vi "YOKOGAWA_CSU-X1.vi"() -> ()   [LabVIEW 2024]
uses:
  States_Ctl.ctl
  <vilib>/Instr/_visa.llb/VISA Flush IO Buffer Mask.ctl
  <vilib>/Instr/_visa.llb/VISA Configure Serial Port (Instr).vi
panel:
  out "YOKOGAWA COM PORT":refnum<visa-resource-name>
  out "Current DM name":string
  out "Current DM position":u16 min=1 max=3 step=1
  out "Current rotation speed":u16=5000 min=1 max=3 step=1
  out "Current filter name 2":string="647LP"
  out "Current Filter position 2":u16=6 min=1 max=3 step=1
  out "Current filter name":string="647LP"
  out "Current Filter position":u16=6 min=1 max=3 step=1
  out "Number of Open/Close":i32=73
  in  "DM names":string[](array[string])=["405488568647", "445514593"]
  in  "DM position":u8=1 min=1 max=2 step=1
  in  "Filter names 2":string[](array[string])=["447BP60", "475BP35", "525BP50", "600BP37", "647BP57", "647LP"]
  in  "FW Position 2":u8=6 min=1 max=6 step=1
  in  "FW Speed 2":u8=3 min=1 max=3 step=1
  in  "Filter names 1":string[](array[string])
  in  "FW Position 1":u8=6 min=1 max=6 step=1
  in  "FW Speed 1":u8=2 min=1 max=3 step=1
  in  "Exposure time (ms)":dbl=50.0 max=5000.0 step=100.0
  in  "Adjust rotation speed\nto exposure time?":bool
  in  "Disk Speed (rpm)":u16=5000 max=0 step=100
  in  "Rotation?":bool=TRUE
  in  "Save dichroic mirror names":bool
  in  "Save filter names":bool
  in  "Shutter":bool
  out "error out":errorcluster
  in  "error in (no error)":errorcluster
  in  "STOP":bool
  # "Disk"
  # "Filter wheel 1"
  # "Filter wheel 2"
  # "Dichroic mirror"
  # "General"
  # "Status"
  # "Advanced settings"
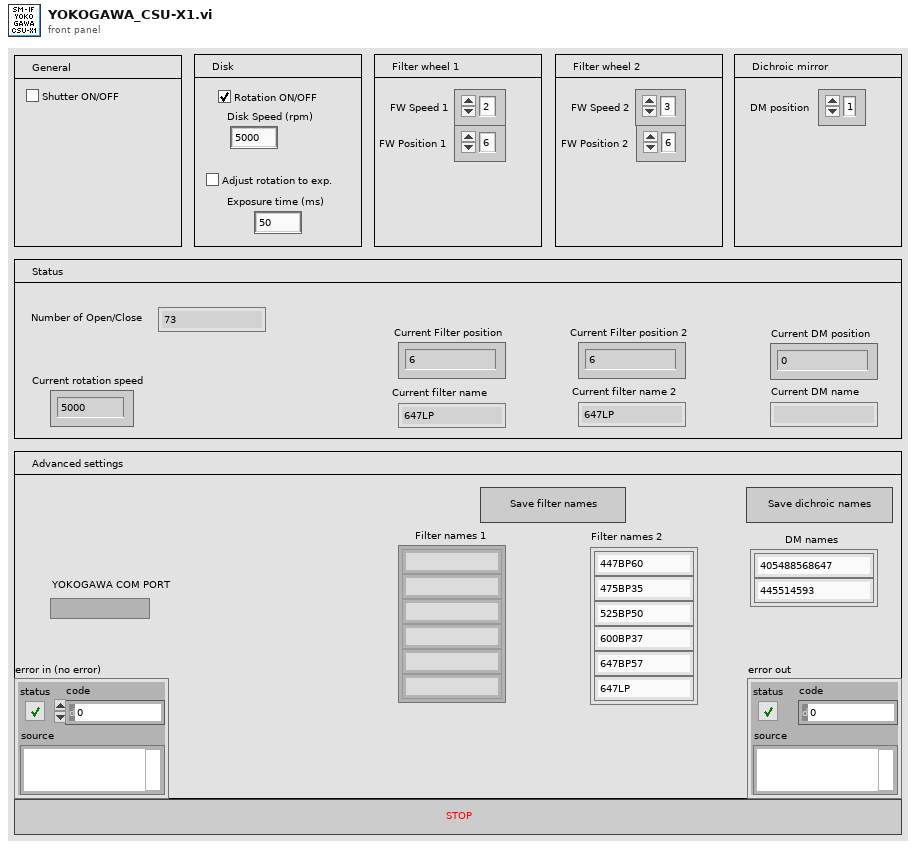
[diagram p1: front panel]
types:
  T1 = typedef "States_Ctl.ctl" = enum16{"INITIALIZE", "WRITE_COMMAND", "CHECK_SHUTTER_STATUS", "CHECK_SHUTTER_COUNT", "CHECK_DISK_SPEED", "CHECK_MAX_DISK_SPEED", "CHECK_FILTER_NAMES", "CHECK_FW_POSITION", "CHECK_DM_POSITION", "CHECK_DM_NAMES", "EXIT"}
  T2 = typedef "VISA Flush IO Buffer Mask.ctl" = u16
  T3 = cluster{"State":T1, "YOKOGAWA COM PORT":refnum<visa-resource-name>}
  T4 = cluster{"State":T1, "Dichroic mirror position":u8}
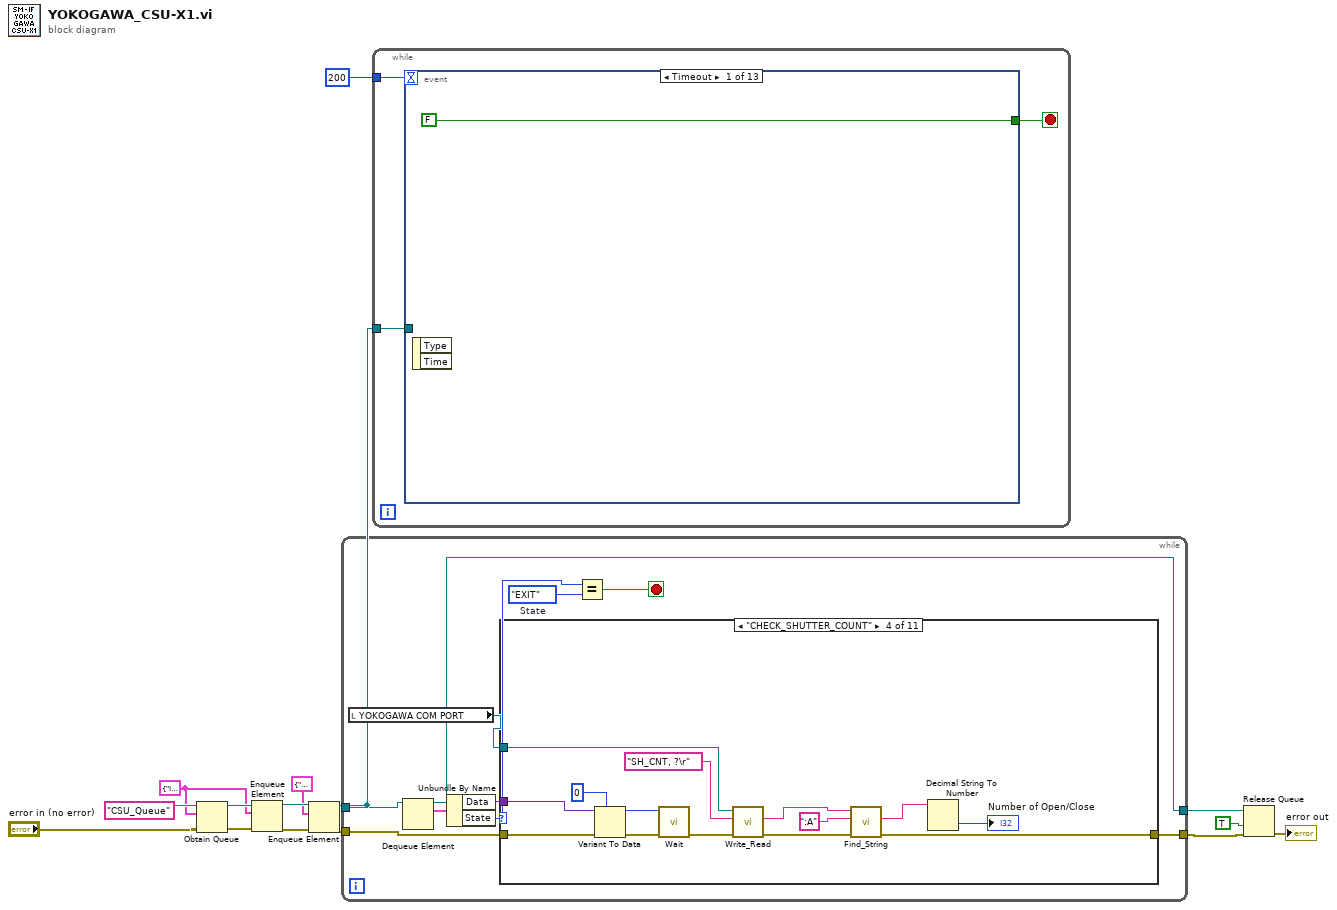
[diagram p0: block diagram]
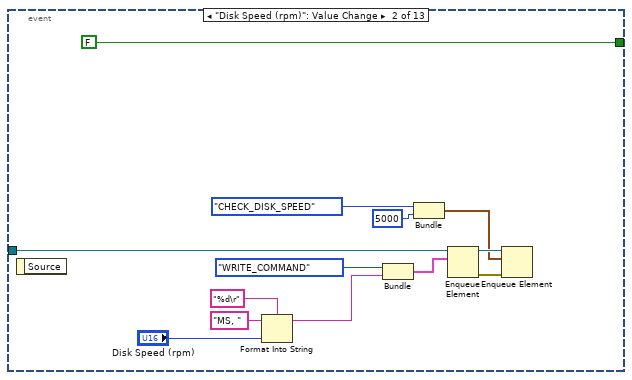
[diagram p2: hidden frame]
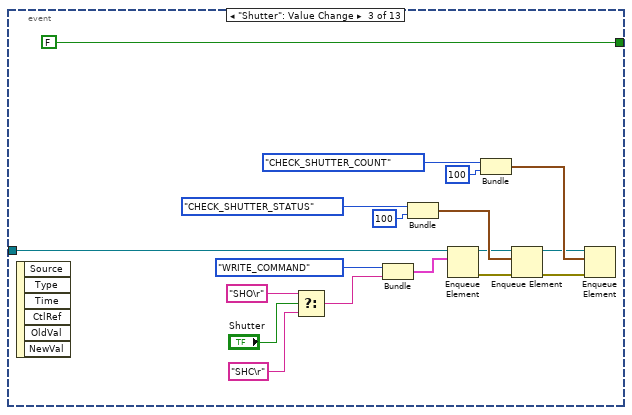
[diagram p3: hidden frame]
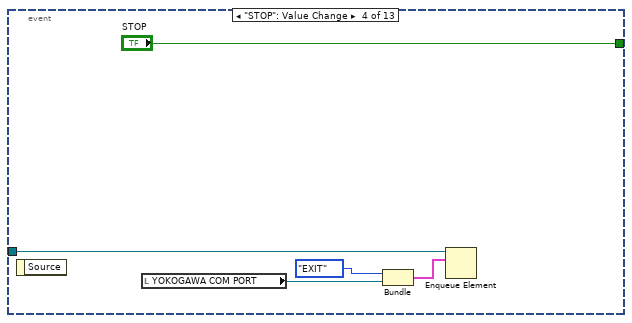
[diagram p4: hidden frame]
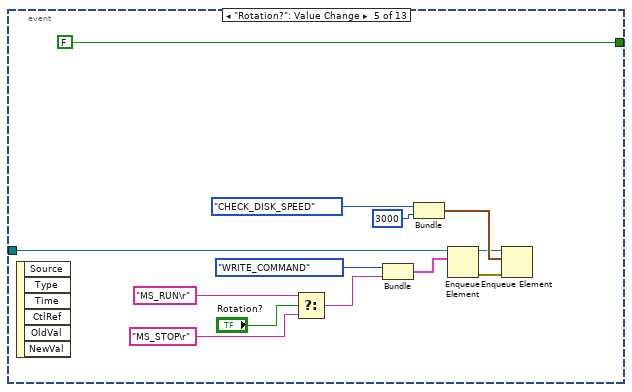
[diagram p5: hidden frame]
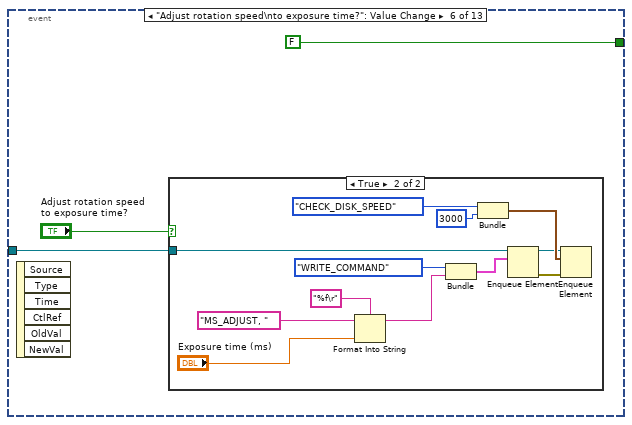
[diagram p6: hidden frame]
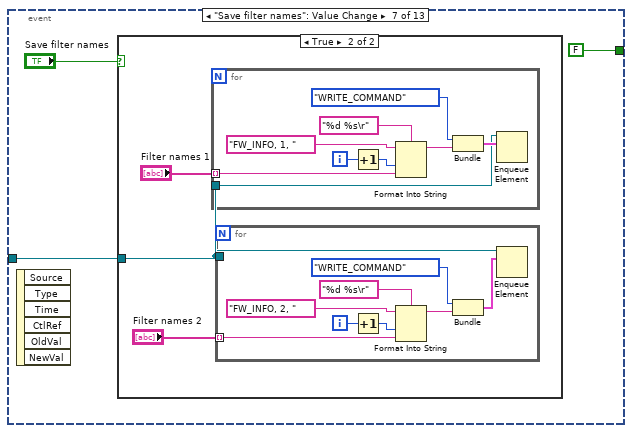
[diagram p8: hidden frame]
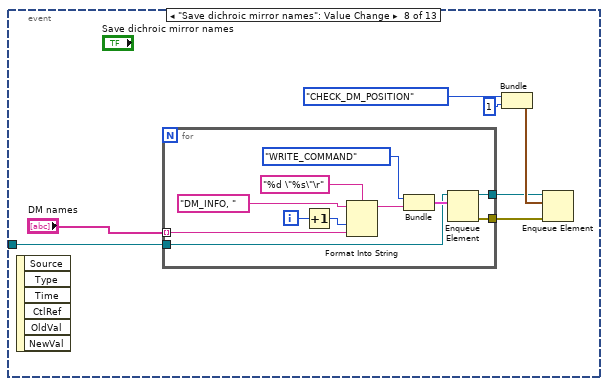
[diagram p10: hidden frame]
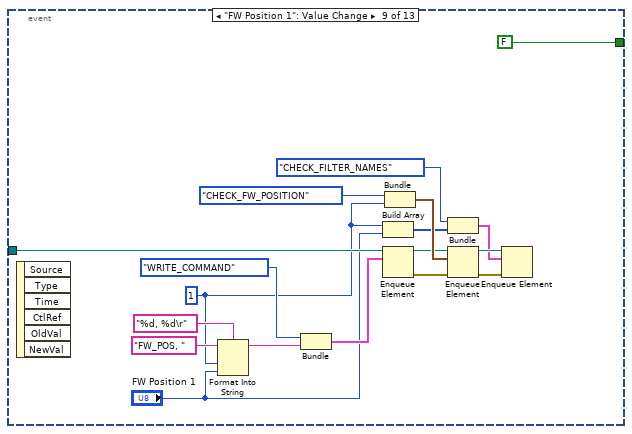
[diagram p11: hidden frame]
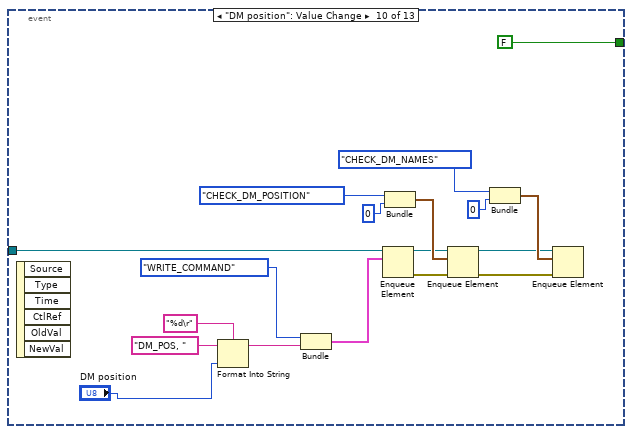
[diagram p12: hidden frame]
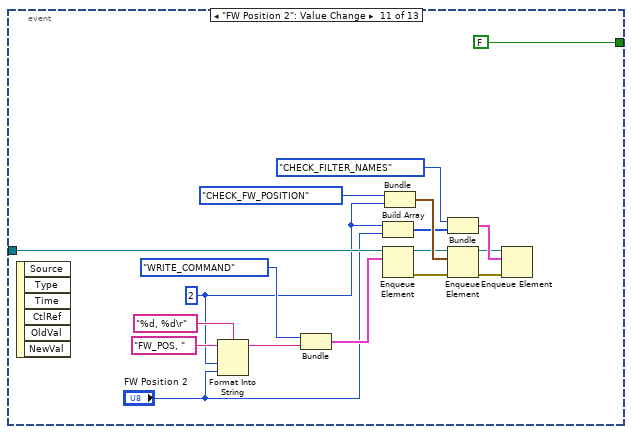
[diagram p13: hidden frame]
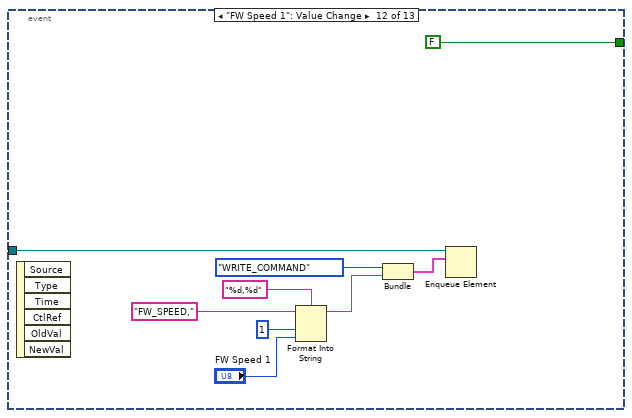
[diagram p14: hidden frame]
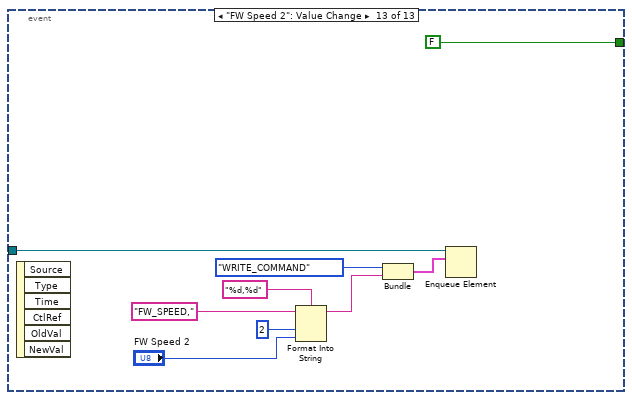
[diagram p15: hidden frame]
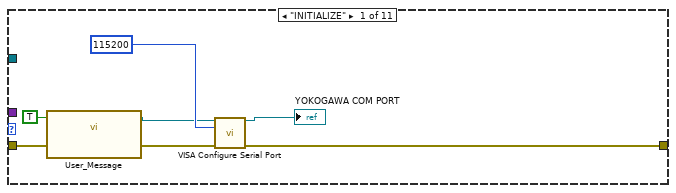
[diagram p16: hidden frame]
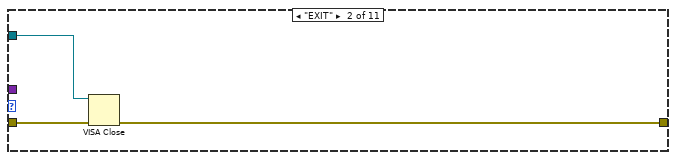
[diagram p17: hidden frame]
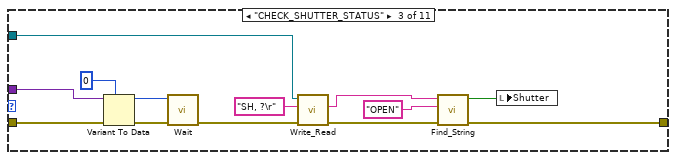
[diagram p18: hidden frame]
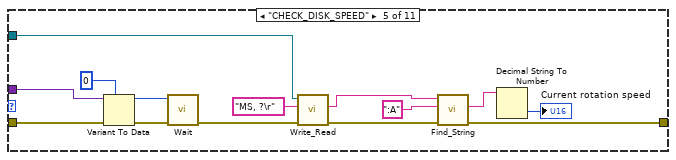
[diagram p19: hidden frame]
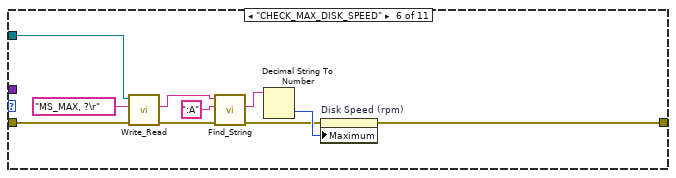
[diagram p20: hidden frame]
diagram:
  w12 = cluster{"State":T1, "Data":variant} {"State"=enum."INITIALIZE", "Data"=variant} ("cluFNData")
  n1 = Obtain Queue(name (unnamed)="CSU_Queue", element data type=w12, error in (no error)="error in (no error)") -> (queue out=w13:refnum<queue>, error out=w14:errorcluster)  [unwired: 2 in, 1 out]
  n2 = Enqueue Element(queue=w13, element=w12, error in (no error)=w14) -> (queue out=w7:refnum<queue>, error out=w8:errorcluster)  [unwired: 1 in, 1 out]
  n3 = Enqueue Element(queue=w7, element=cluster{"State":T1, "Data":variant} {"State"=enum."CHECK_MAX_DISK_SPEED", "Data"=variant} ("cluFNData"), error in (no error)=w8) -> (queue out=w1:refnum<queue>, error out=w5:errorcluster)  [unwired: 1 in, 1 out]
  n4 = while {
    tunnel: w5 -> [w21]
    tunnel: w1 -> [w20]
    tunnel: [w19] -> w4
    tunnel: [w18] -> w3
    stop <- w17 stop-if-true
    w22 = States_Ctl."EXIT"  # State
    n5 = local read "YOKOGAWA COM PORT"() -> (w16:refnum<visa-resource-name>)
    n6 = Dequeue Element(queue=w20) -> (queue out=w19:refnum<queue>, element=w23:cluster{"State":T1, "Data":variant})  [unwired: 2 in, 2 out]
    n7 = Unbundle By Name(w23) -> ("Data"=w24:variant, "State"=w25:T1)
    n8 = case shown="\"CHECK_SHUTTER_COUNT\"" w25 {
      tunnel: w21 -> [w30 w34 w37 w50 w65 w81 w91 w108 w123 w150 w156]
      tunnel: [w31 w35 w43 w56 w71 w77 w92 w102 w128 w137 w158] -> w18
      tunnel: w24 -> [_ _ w36 w51 w64 _ w94 w109 _ w151 _]
      tunnel: w16 -> [_ w33 w42 w57 w69 w80 w90 w110 w121 w142 w157]
      frame "INITIALIZE" {
        n9 = call "User_Message.vi"("Enable"=TRUE, "error in (no error)"=w30) -> ("CSU COM PORT  2"=w26:refnum<visa-resource-name>, "error out"=w28:errorcluster)  [unwired: 15 in, 1 out]
        n10 = call-poly "VISA Configure Serial Port"("VISA resource name"=w26, "baud rate (9600)"=u32 115200, "error in (no error)"=w28) -> ("VISA resource name out"=→"YOKOGAWA COM PORT":refnum<visa-resource-name>, "error out"=w31:errorcluster)  [unwired: 11 in]
      }
      frame "EXIT" {
        n11 = VISA Close(VISA resource name=w33, error in (no error)=w34) -> (error out=w35:errorcluster)
      }
      frame "CHECK_SHUTTER_STATUS" {
        n12 = Variant To Data(error in=w37, type=0, Variant=w36) -> (data=w40:i32, error out=w39:errorcluster)
        n13 = call "Wait.vi"("error in (no error)"=w39, "milliseconds to wait"=w40) -> ("error out"=w38:errorcluster)  [unwired: 9 in]
        n14 = call "Write_Read.vi"("error in (no error)"=w38, "String"="SH, ?\r", "VISA Refnum in"=w42) -> ("error out"=w45:errorcluster, "Response"=w47:string)  [unwired: 6 in, 1 out]
        n15 = call "Find_String.vi"("error in"=w45, "String to find"="OPEN" ("Response"), "Input string"=w47) -> ("error out"=w43:errorcluster, "Found?"=w44:bool)  [unwired: 5 in, 2 out]
        n16 = local write "Shutter"(w44) -> ()
      }
      frame "CHECK_SHUTTER_COUNT" {
        n17 = Variant To Data(error in=w50, type=0, Variant=w51) -> (data=w54:i32, error out=w53:errorcluster)
        n18 = call "Wait.vi"("error in (no error)"=w53, "milliseconds to wait"=w54) -> ("error out"=w49:errorcluster)  [unwired: 9 in]
        n19 = call "Write_Read.vi"("error in (no error)"=w49, "String"="SH_CNT, ?\r", "VISA Refnum in"=w57) -> ("error out"=w60:errorcluster, "Response"=w61:string)  [unwired: 6 in, 1 out]
        n20 = call "Find_String.vi"("error in"=w60, "String to find"=":A", "Input string"=w61) -> ("error out"=w56:errorcluster, "before substring"=w62:string)  [unwired: 5 in, 2 out]
        n21 = Decimal String To Number(string=w62) -> (number=→"Number of Open/Close":i32)  [unwired: 2 in, 1 out]
      }
      frame "CHECK_DISK_SPEED" {
        n22 = Variant To Data(error in=w65, type=0, Variant=w64) -> (data=w67:i32, error out=w68:errorcluster)
        n23 = call "Wait.vi"("error in (no error)"=w68, "milliseconds to wait"=w67) -> ("error out"=w63:errorcluster)  [unwired: 9 in]
        n24 = call "Write_Read.vi"("error in (no error)"=w63, "String"="MS, ?\r" ("string"), "VISA Refnum in"=w69) -> ("error out"=w73:errorcluster, "Response"=w74:string)  [unwired: 6 in, 1 out]
        n25 = call "Find_String.vi"("error in"=w73, "String to find"=":A", "Input string"=w74) -> ("error out"=w71:errorcluster, "before substring"=w76:string)  [unwired: 5 in, 2 out]
        n26 = Decimal String To Number(string=w76) -> (number=→"Current rotation speed":i32)  [unwired: 2 in, 1 out]
      }
      frame "CHECK_MAX_DISK_SPEED" {
        n27 = call "Write_Read.vi"("error in (no error)"=w81, "String"="MS_MAX, ?\r" ("string"), "VISA Refnum in"=w80) -> ("error out"=w83:errorcluster, "Response"=w84:string)  [unwired: 6 in, 1 out]
        n28 = call "Find_String.vi"("error in"=w83, "String to find"=":A", "Input string"=w84) -> ("error out"=w78:errorcluster, "before substring"=w86:string)  [unwired: 5 in, 2 out]
        n29 = Decimal String To Number(string=w86) -> (number=w79:i32)  [unwired: 2 in, 1 out]
        n30 = property on="Disk Speed (rpm)" class="DigNum (strict)"(error in=w78, "Maximum"=w79) -> (error out=w77:errorcluster)  [unwired: 1 in, 1 out]
      }
      frame "WRITE_COMMAND" {
        w87 = T2 16 items=["Flush Receive Buffer"=16, "Write Transmit Buffer to Device"=32, "Flush Receive Buffer (No I/O)"=64, "Flush Transmit Buffer"=128] ("Mask")
        n31 = VISA Flush I/O Buffer(VISA resource name=w90, mask (16)=w87, error in (no error)=w91) -> (VISA resource name out=w88:refnum<visa-resource-name>, error out=w89:errorcluster)
        n32 = Variant To Data(error in=w89, type="", Variant=w94) -> (data=w93:string, error out=w96:errorcluster)
        n33 = call "Write_Read.vi"("error in (no error)"=w96, "String"=w93, "VISA Refnum in"=w88) -> ("error out"=w92:errorcluster)  [unwired: 6 in, 2 out]
      }
      frame "CHECK_FW_POSITION" {
        n34 = Variant To Data(error in=w108, type=u8 1 ("input 1"), Variant=w109) -> (data=w101:u8, error out=w103:errorcluster)
        n35 = Equal?(x=u8 1, y=w101) -> (x = y?=w99:bool)
        n36 = Format Into String(format string="%d, ?\r", initial string="FW_POS, " ("string"), w101) -> (resulting string=w104:string)  [unwired: 1 in, 1 out]
        n37 = call "Write_Read.vi"("delay before read (ms)"=u32 50, "error in (no error)"=w103, "String"=w104, "VISA Refnum in"=w110) -> ("error out"=w111:errorcluster, "Response"=w112:string)  [unwired: 5 in, 1 out]
        n38 = call "Find_String.vi"("error in"=w111, "String to find"=":A", "Input string"=w112) -> ("error out"=w102:errorcluster, "before substring"=w114:string)  [unwired: 5 in, 2 out]
        n39 = Decimal String To Number(string=w114) -> (number=w97:i32)  [unwired: 2 in, 1 out]
        n40 = case shown="True" w99 {
          tunnel: w97 -> [w115 w116]
          frame False {
            "Current Filter position 2" <- w115
          }
          frame True {
            "Current Filter position" <- w116
          }
        }
      }
      frame "CHECK_DM_POSITION" {
        w117 = T2 16 items=["Flush Receive Buffer"=16, "Write Transmit Buffer to Device"=32, "Flush Receive Buffer (No I/O)"=64, "Flush Transmit Buffer"=128] ("Mask")
        n41 = call "Wait.vi"("error in (no error)"=w123, "milliseconds to wait"=u32 1000) -> ("error out"=w120:errorcluster)  [unwired: 9 in]
        n42 = VISA Flush I/O Buffer(VISA resource name=w121, mask (16)=w117, error in (no error)=w120) -> (VISA resource name out=w118:refnum<visa-resource-name>, error out=w119:errorcluster)
        n43 = call "Write_Read.vi"("delay before read (ms)"=u32 50, "error in (no error)"=w119, "String"="DM_POS, ?\r" ("Command"), "VISA Refnum in"=w118) -> ("error out"=w129:errorcluster, "Response"=w130:string)  [unwired: 5 in, 1 out]
        n44 = call "Find_String.vi"("error in"=w129, "String to find"=":A", "Input string"=w130) -> ("error out"=w128:errorcluster, "before substring"=w126:string)  [unwired: 5 in, 2 out]
        n45 = Decimal String To Number(string=w126) -> (number=→"Current DM position":i32)  [unwired: 2 in, 1 out]
      }
      frame "CHECK_FILTER_NAMES" {
        n46 = Variant To Data(error in=w150, type=u8[] [2, 3] ("appended array 2"), Variant=w151) -> (data=w144:u8[], error out=w132:errorcluster)
        n47 = Index Array(array=w144, index=0) -> (element=w135:u8)
        n48 = Index Array(array=w144, index=1) -> (element=w143:u8)
        n49 = Format Into String(format string="%d, %d,\\s?\\r", initial string="FW_INFO, " ("string"), w135, w143) -> (resulting string=w141:string)  [unwired: 1 in, 1 out]
        n50 = Equal?(x=u8 1, y=w135) -> (x = y?=w134:bool)
        n51 = call "Write_Read.vi"("error in (no error)"=w132, "String"=w141, "VISA Refnum in"=w142) -> ("error out"=w138:errorcluster, "Response"=w140:string)  [unwired: 6 in, 1 out]
        n52 = call "Find_String.vi"("error in"=w138, "String to find"=":A", "Input string"=w140) -> ("error out"=w137:errorcluster, "before substring"=w133:string)  [unwired: 5 in, 2 out]
        n53 = case shown="False" w134 {
          tunnel: w133 -> [w152 w153]
          frame False {
            "Current filter name 2" <- w152
          }
          frame True {
            "Current filter name" <- w153
          }
        }
      }
      frame "CHECK_DM_NAMES" {
        w154 = T2 16 items=["Flush Receive Buffer"=16, "Write Transmit Buffer to Device"=32, "Flush Receive Buffer (No I/O)"=64, "Flush Transmit Buffer"=128] ("Mask")
        n54 = local read "Current DM position"() -> (w167:u16)
        n55 = VISA Flush I/O Buffer(VISA resource name=w157, mask (16)=w154, error in (no error)=w156) -> (error out=w155:errorcluster)  [unwired: 1 out]
        n56 = Format Into String(format string="%d,\\s?\\r", initial string="DM_INFO, " ("string"), error in=w155, w167) -> (resulting string=w168:string, error out=w159:errorcluster)
        n57 = call "Write_Read.vi"("delay before read (ms)"=u32 50, "error in (no error)"=w159, "String"=w168, "VISA Refnum in"=w157) -> ("error out"=w162:errorcluster, "Response"=w161:string)  [unwired: 5 in, 1 out]
        n58 = call "Find_String.vi"("error in"=w162, "String to find"=":A", "Input string"=w161) -> ("error out"=w158:errorcluster, "before substring"=→"Current DM name":string)  [unwired: 5 in, 2 out]
      }
    }
    n59 = Equal?(x=w25, y=w22) -> (x = y?=w17:bool)
  }
  n60 = while {
    tunnel: 200 -> [w171]
    tunnel: w1 -> [w170]
    stop <- w169 stop-if-true
    n61 = event shown="[0] Timeout" {
      selector: _ -> [_ _ _ _ _ _ _ _ _ _ _ _ _]
      dyn-events: _ -> [_ _ _ _ _ _ _ _ _ _ _ _ _]
      timeout: w171 -> [_ _ _ _ _ _ _ _ _ _ _ _ _]
      tunnel: w170 -> [_ w182 w200 w208 w214 w223 w238 w266 w294 w312 w330 w336 w345]
      tunnel: [FALSE ("STOP") FALSE ("STOP") FALSE ("STOP") "STOP" FALSE ("STOP") FALSE ("STOP") FALSE ("STOP") _ FALSE ("STOP") FALSE ("STOP") FALSE ("STOP") FALSE ("STOP") FALSE ("STOP")] -> w169
      event Timeout {
        n62 = event-data() -> ()  [unwired: 1 in, 2 out]
      }
      event "Disk Speed (rpm)": Value Change {
        n63 = event-data() -> ()  [unwired: 1 in, 1 out]
        n64 = Format Into String(format string="%d\r", initial string="MS, ", "Disk Speed (rpm)") -> (resulting string=w178:string)  [unwired: 1 in, 1 out]
        n65 = Bundle("State"=States_Ctl."WRITE_COMMAND", w178) -> (w183:cluster{"State":T1, string})  [unwired: 1 in]
        n66 = Bundle("State"=States_Ctl."CHECK_DISK_SPEED", 5000) -> (w173:cluster{"State":T1, i32})  [unwired: 1 in]
        n67 = Enqueue Element(queue=w182, element=w183) -> (queue out=w176:refnum<queue>, error out=w177:errorcluster)  [unwired: 2 in, 1 out]
        n68 = Enqueue Element(queue=w176, element=w173, error in (no error)=w177) -> ()  [unwired: 1 in, 3 out]
      }
      event "Shutter": Value Change {
        n69 = event-data() -> ()  [unwired: 1 in, 6 out]
        n70 = Select(t="SHO\r", s="Shutter", f="SHC\r") -> (s? t:f=w196:string)
        n71 = Bundle("State"=States_Ctl."WRITE_COMMAND", w196) -> (w202:cluster{"State":T1, string})  [unwired: 1 in]
        n72 = Bundle("State"=States_Ctl."CHECK_SHUTTER_STATUS", 100) -> (w195:cluster{"State":T1, i32})  [unwired: 1 in]
        n73 = Enqueue Element(queue=w200, element=w202) -> (queue out=w193:refnum<queue>, error out=w186:errorcluster)  [unwired: 2 in, 1 out]
        n74 = Bundle("State"=States_Ctl."CHECK_SHUTTER_COUNT", 100) -> (w191:cluster{"State":T1, i32})  [unwired: 1 in]
        n75 = Enqueue Element(queue=w193, element=w195, error in (no error)=w186) -> (queue out=w188:refnum<queue>, error out=w187:errorcluster)  [unwired: 1 in, 1 out]
        n76 = Enqueue Element(queue=w188, element=w191, error in (no error)=w187) -> ()  [unwired: 1 in, 3 out]
      }
      event "STOP": Value Change {
        n77 = event-data() -> ()  [unwired: 1 in, 1 out]
        n78 = local read "YOKOGAWA COM PORT"() -> (w204:refnum<visa-resource-name>)
        n79 = Bundle("State"=States_Ctl."EXIT", "YOKOGAWA COM PORT"=w204) -> (w206:T3)  [unwired: 1 in]
        n80 = Enqueue Element(queue=w208, element=w206) -> ()  [unwired: 2 in, 3 out]
      }
      event "Rotation?": Value Change {
        n81 = event-data() -> ()  [unwired: 1 in, 6 out]
        n82 = Select(t="MS_RUN\r", s="Rotation?", f="MS_STOP\r") -> (s? t:f=w215:string)
        n83 = Bundle("State"=States_Ctl."WRITE_COMMAND", w215) -> (w217:cluster{"State":T1, string})  [unwired: 1 in]
        n84 = Bundle("State"=States_Ctl."CHECK_DISK_SPEED", 3000) -> (w213:cluster{"State":T1, i32})  [unwired: 1 in]
        n85 = Enqueue Element(queue=w214, element=w217) -> (queue out=w211:refnum<queue>, error out=w210:errorcluster)  [unwired: 2 in, 1 out]
        n86 = Enqueue Element(queue=w211, element=w213, error in (no error)=w210) -> ()  [unwired: 1 in, 3 out]
      }
      event "Adjust rotation speed\nto exposure time?": Value Change {
        n87 = event-data() -> ()  [unwired: 1 in, 6 out]
        n88 = case shown="True" "Adjust rotation speed\nto exposure time?" {
          tunnel: w223 -> [_ w234]
          frame False {
          }
          frame True {
            n89 = Format Into String(format string="%f\r", initial string="MS_ADJUST, ", "Exposure time (ms)") -> (resulting string=w230:string)  [unwired: 1 in, 1 out]
            n90 = Bundle("State"=States_Ctl."WRITE_COMMAND", w230) -> (w235:cluster{"State":T1, string})  [unwired: 1 in]
            n91 = Bundle("State"=States_Ctl."CHECK_DISK_SPEED", "Exposure time (ms)"=u16 3000) -> (w229:cluster{"State":T1, "Exposure time (ms)":u16})  [unwired: 1 in]
            n92 = Enqueue Element(queue=w234, element=w235) -> (queue out=w227:refnum<queue>, error out=w226:errorcluster)  [unwired: 2 in, 1 out]
            n93 = Enqueue Element(queue=w227, element=w229, error in (no error)=w226) -> ()  [unwired: 1 in, 3 out]
          }
        }
      }
      event "Save filter names": Value Change {
        n94 = event-data() -> ()  [unwired: 1 in, 6 out]
        n95 = case shown="True" "Save filter names" {
          tunnel: w238 -> [_ w241]
          frame False {
          }
          frame True {
            n96 = for {
              tunnel: "Filter names 1" -> [w255] mode=indexing
              tunnel: w241 -> [w253]
              i -> [w257]
              n97 = Increment(x=w257) -> (x+1=w256:i32)
              n98 = Format Into String(format string="%d %s\r", initial string="FW_INFO, 1, ", w256, w255) -> (resulting string=w254:string)  [unwired: 1 in, 1 out]
              n99 = Bundle("State"=States_Ctl."WRITE_COMMAND", w254) -> (w260:cluster{"State":T1, string})  [unwired: 1 in]
              n100 = Enqueue Element(queue=w253, element=w260) -> ()  [unwired: 2 in, 3 out]
            }
            n101 = for {
              tunnel: "Filter names 2" -> [w246] mode=indexing
              tunnel: w241 -> [w244]
              i -> [w248]
              n102 = Increment(x=w248) -> (x+1=w247:i32)
              n103 = Format Into String(format string="%d %s\r", initial string="FW_INFO, 2, ", w247, w246) -> (resulting string=w245:string)  [unwired: 1 in, 1 out]
              n104 = Bundle("State"=States_Ctl."WRITE_COMMAND", w245) -> (w251:cluster{"State":T1, string})  [unwired: 1 in]
              n105 = Enqueue Element(queue=w244, element=w251) -> ()  [unwired: 2 in, 3 out]
            }
          }
        }
      }
      event "Save dichroic mirror names": Value Change {
        n106 = event-data() -> ()  [unwired: 1 in, 6 out]
        n107 = for {
          tunnel: "DM names" -> [w273] mode=indexing
          tunnel: w266 -> [w271]
          tunnel: [w269] -> w263
          tunnel: [w268] -> w261
          i -> [w275]
          n108 = Increment(x=w275) -> (x+1=w274:i32)
          n109 = Format Into String(format string="%d \"%s\"\r", initial string="DM_INFO, ", w274, w273) -> (resulting string=w272:string)  [unwired: 1 in, 1 out]
          n110 = Bundle("State"=States_Ctl."WRITE_COMMAND", w272) -> (w278:cluster{"State":T1, string})  [unwired: 1 in]
          n111 = Enqueue Element(queue=w271, element=w278) -> (queue out=w268:refnum<queue>, error out=w269:errorcluster)  [unwired: 2 in, 1 out]
        }
        n112 = Bundle("State"=States_Ctl."CHECK_DM_POSITION", "x+1"=1) -> (w264:cluster{"State":T1, "x+1":i32})  [unwired: 1 in]
        n113 = Enqueue Element(queue=w261, element=w264, error in (no error)=w263) -> ()  [unwired: 1 in, 3 out]
      }
      event "FW Position 1": Value Change {
        w283 = u8 1 ("input 1")
        n114 = event-data() -> ()  [unwired: 1 in, 6 out]
        n115 = Format Into String(format string="%d, %d\r", initial string="FW_POS, ", w283, "FW Position 1") -> (resulting string=w291:string)  [unwired: 1 in, 1 out]
        n116 = Bundle("State"=States_Ctl."WRITE_COMMAND", w291) -> (w295:cluster{"State":T1, string})  [unwired: 1 in]
        n117 = Build Array(w283, "FW Position 1") -> (w284:u8[])
        n118 = Enqueue Element(queue=w294, element=w295) -> (queue out=w286:refnum<queue>, error out=w287:errorcluster)  [unwired: 2 in, 1 out]
        n119 = Bundle("State"=States_Ctl."CHECK_FW_POSITION", "input 1"=w283) -> (w289:cluster{"State":T1, "input 1":u8})  [unwired: 1 in]
        n120 = Bundle("State"=States_Ctl."CHECK_FILTER_NAMES", w284) -> (w279:cluster{"State":T1, u8[]})  [unwired: 1 in]
        n121 = Enqueue Element(queue=w286, element=w289, error in (no error)=w287) -> (queue out=w280:refnum<queue>, error out=w281:errorcluster)  [unwired: 1 in, 1 out]
        n122 = Enqueue Element(queue=w280, element=w279, error in (no error)=w281) -> ()  [unwired: 1 in, 3 out]
      }
      event "DM position": Value Change {
        n123 = event-data() -> ()  [unwired: 1 in, 6 out]
        n124 = Format Into String(format string="%d\r", initial string="DM_POS, ", "DM position") -> (resulting string=w309:string)  [unwired: 1 in, 1 out]
        n125 = Bundle("State"=States_Ctl."WRITE_COMMAND", w309) -> (w313:cluster{"State":T1, string})  [unwired: 1 in]
        n126 = Enqueue Element(queue=w312, element=w313) -> (queue out=w304:refnum<queue>, error out=w305:errorcluster)  [unwired: 2 in, 1 out]
        n127 = Bundle("State"=States_Ctl."CHECK_DM_POSITION", "Dichroic mirror position"=u8 0) -> (w307:T4)  [unwired: 1 in]
        n128 = Enqueue Element(queue=w304, element=w307, error in (no error)=w305) -> (queue out=w298:refnum<queue>, error out=w297:errorcluster)  [unwired: 1 in, 1 out]
        n129 = Bundle("State"=States_Ctl."CHECK_DM_NAMES", "Dichroic mirror position"=u8 0) -> (w301:T4)  [unwired: 1 in]
        n130 = Enqueue Element(queue=w298, element=w301, error in (no error)=w297) -> ()  [unwired: 1 in, 3 out]
      }
      event "FW Position 2": Value Change {
        w317 = u8 2 ("input 1")
        n131 = event-data() -> ()  [unwired: 1 in, 6 out]
        n132 = Format Into String(format string="%d, %d\r", initial string="FW_POS, ", w317, "FW Position 2") -> (resulting string=w327:string)  [unwired: 1 in, 1 out]
        n133 = Bundle("State"=States_Ctl."WRITE_COMMAND", w327) -> (w331:cluster{"State":T1, string})  [unwired: 1 in]
        n134 = Build Array(w317, "FW Position 2") -> (w315:u8[])
        n135 = Enqueue Element(queue=w330, element=w331) -> (queue out=w323:refnum<queue>, error out=w322:errorcluster)  [unwired: 2 in, 1 out]
        n136 = Bundle("State"=States_Ctl."CHECK_FW_POSITION", "input 1"=w317) -> (w324:cluster{"State":T1, "input 1":u8})  [unwired: 1 in]
        n137 = Bundle("State"=States_Ctl."CHECK_FILTER_NAMES", w315) -> (w321:cluster{"State":T1, u8[]})  [unwired: 1 in]
        n138 = Enqueue Element(queue=w323, element=w324, error in (no error)=w322) -> (queue out=w319:refnum<queue>, error out=w318:errorcluster)  [unwired: 1 in, 1 out]
        n139 = Enqueue Element(queue=w319, element=w321, error in (no error)=w318) -> ()  [unwired: 1 in, 3 out]
      }
      event "FW Speed 1": Value Change {
        n140 = event-data() -> ()  [unwired: 1 in, 6 out]
        n141 = Format Into String(format string="%d,%d", initial string="FW_SPEED,", u8 1 ("input 1"), "FW Speed 1") -> (resulting string=w337:string)  [unwired: 1 in, 1 out]
        n142 = Bundle("State"=States_Ctl."WRITE_COMMAND", w337) -> (w338:cluster{"State":T1, string})  [unwired: 1 in]
        n143 = Enqueue Element(queue=w336, element=w338) -> ()  [unwired: 2 in, 3 out]
      }
      event "FW Speed 2": Value Change {
        n144 = event-data() -> ()  [unwired: 1 in, 6 out]
        n145 = Format Into String(format string="%d,%d", initial string="FW_SPEED,", u8 2 ("input 1"), "FW Speed 2") -> (resulting string=w346:string)  [unwired: 1 in, 1 out]
        n146 = Bundle("State"=States_Ctl."WRITE_COMMAND", w346) -> (w347:cluster{"State":T1, string})  [unwired: 1 in]
        n147 = Enqueue Element(queue=w345, element=w347) -> ()  [unwired: 2 in, 3 out]
      }
    }
  }
  n148 = Release Queue(queue=w4, force destroy? (F)=TRUE, error in (no error)=w3) -> (error out=→"error out":errorcluster)  [unwired: 2 out]
